vi "IMULoop.vi"   [LabVIEW 2015]
uses:
  Common Code/IMU Data.ctl
  Robot Global Data.vi
  navX-MXP Library/navX-MXP IMU.lvlib
  navX.Library.v2/navX Library v2/navX Library v2.lvlib
  navX.Library.v2/navX Library v2/TypeDefs/Flags/Z900_navX_Flags_OpStatusTypeDef.ctl
  navX.Library.v2/navX Library v2/TypeDefs/Flags/Z900_navX_Flags_CalibrationStatusTypeDef.ctl
types:
  T1 = typedef "IMU Data.ctl" = cluster{"Pitch":sgl, "Roll":sgl, "Yaw":sgl, "Data Valid?":bool, "Temp":sgl, "MOVING":bool, "YAW_STABLE":bool, "Accel X":sgl, "Accel Y":sgl, "Accel Z":sgl, "Accel Magnitude":sgl, "Pitch Rate":sgl, "Roll Rate":sgl, "Yaw Rate":sgl, "NavX Opened?":bool, "Calibration Status":T2, "OP Status":T3}
  T2 = typedef "navX Library v2.lvlib/Z900_navX_Flags_CalibrationStatusTypeDef.ctl" = u8
  T3 = typedef "navX Library v2.lvlib/Z900_navX_Flags_OpStatusTypeDef.ctl" = u8
  T4 = typedef "navX-MXP IMU.lvlib/navX Device TypeDef.ctl" = cluster{"navX Interface Protocol":T5, "navX Interface Protocol TypeDefs":cluster{"SPIDevRef":T6, "I2CDevRef":T8}, "navX System Information":cluster{"Board Information":T10, "Status":T11, "Offsets":T15}, "navX Common Information":cluster{"Update Rate (4Hz-60Hz)":T16, "refnum name":string, "error":errorcluster}}
  T5 = typedef "navX-MXP IMU.lvlib/navX Interface Protocol.ctl" = enum16{"SPI", "I2C"}
  T6 = typedef "WPI_SPIDevRef.ctl" = cluster{"DevStatus":errorcluster, "Handle":i32, "SPI Bus":T7}
  T7 = typedef "spi_bus.ctl" = enum16{"SPI On-Board, CS0", "SPI On-Board, CS1", "SPI On-Board, CS2", "SPI On-Board, CS3", "SPI MXP", "Invalid"}
  T8 = typedef "WPI_I2CDevRef.ctl" = cluster{"DevStatus":errorcluster, "Device Address":u8, "Handle":i32, "I2C Bus":T9}
  T9 = typedef "i2c_bus.ctl" = enum16{"I2C On-Board", "I2C MXP", "Invalid"}
  T10 = typedef "navX-MXP IMU.lvlib/navX Board Information.ctl" = cluster{"WhoAmI (50 | 0x32)":u8, "Board Revision":u8, "Firmware Major Version":u8, "Firmware Minor Version":u8}
  T11 = typedef "navX-MXP IMU.lvlib/navX Status Data.ctl" = cluster{"Update Rate Hz":u8, "Accelerometer Full-Scale Range":u8, "Gyro Full-Scale Range":u16, "NAVX_OP_STATUS":T12, "NAVX_CAL_STATUS":T13, "NAVX_SELFTEST_STATUS":u8, "NAVX_SENSOR_STATUS":T14}
  T12 = typedef "navX-MXP IMU.lvlib/navX NAVX_OP_STATUS.ctl" = u8
  T13 = typedef "navX-MXP IMU.lvlib/navX NAVX_CAL_STATUS.ctl" = u8
  T14 = typedef "navX-MXP IMU.lvlib/navX NAVX_SENSOR_STATUS.ctl" = cluster{"MOVING":bool, "YAW_STABLE":bool, "MAG_DISTURBANCE":bool, "ALTITUDE_VALID":bool, "SEALEVEL_PRESS_SET":bool, "FUSED_HEADING_VALID":bool}
  T15 = typedef "navX-MXP IMU.lvlib/navX Offsets Data.ctl" = cluster{"Yaw":dbl, "Quat W":dbl, "Quat X":dbl, "Quat Y":dbl, "Quat Z":dbl}
  T16 = typedef "navX-MXP IMU.lvlib/navX Update Rate.ctl" = u8
  T17 = typedef "navX-MXP IMU.lvlib/navX Vector Data.ctl" = cluster{"X":dbl, "Y":dbl, "Z":dbl}
  T18 = typedef "navX-MXP IMU.lvlib/navX YPRH Data.ctl" = cluster{"Yaw":dbl, "Pitch":dbl, "Roll":dbl, "Heading":dbl}
  T19 = typedef "navX Library v2.lvlib/Z900_navX_DeviceTypeDef.ctl" = cluster{"Interface":cluster{"Protocol":T20, "Update Rate (4Hz-60Hz)":u8, "navX Open TypeDef":variant}, "Notify Packet":refnum<notifier>, "Loop VI Refnum":refnum<vi>, "Ready to Close Occurrence Refnum":refnum<k4>}
  T20 = typedef "navX Library v2.lvlib/Z900_navX_ProtocolTypeDef.ctl" = enum16{"SERIAL", "I2C", "SPI"}
  T21 = cluster{"Accel X":dbl, "Accel Y":dbl, "Accel Z":dbl, "Gyro X":dbl, "Gyro Y":dbl, "Gyro Z":dbl, "Mag X":dbl, "Mag Y":dbl, "Mag Z":dbl}
  T22 = cluster{"Yaw":dbl, "Roll":dbl, "Pitch":dbl, "Heading":dbl, "Fused Heading":dbl}
  T23 = cluster{"Update Rate Hz":u8, "Accelerometer Full-Scale Range":u8, "Gyro Full-Scale Range":u16, "OP Status":T3, "Calibration Status":T2, "Sensor Status":cluster{"MOVING":bool, "YAW_STABLE":bool, "MAG_DISTURBANCE":bool, "ALTITUDE_VALID":bool, "SEALEVEL_PRESS_SET":bool, "FUSED_HEADING_VALID":bool}, "Self Test Status":cluster{"Gyro Passed":bool, "Accel Passed":bool, "Mag Passed":bool, "Baro Passed":bool, "Complete":bool}}
  T24 = cluster{"LinearAcceleration X":dbl, "LinearAcceleration Y":dbl, "LinearAcceleration Z":dbl}
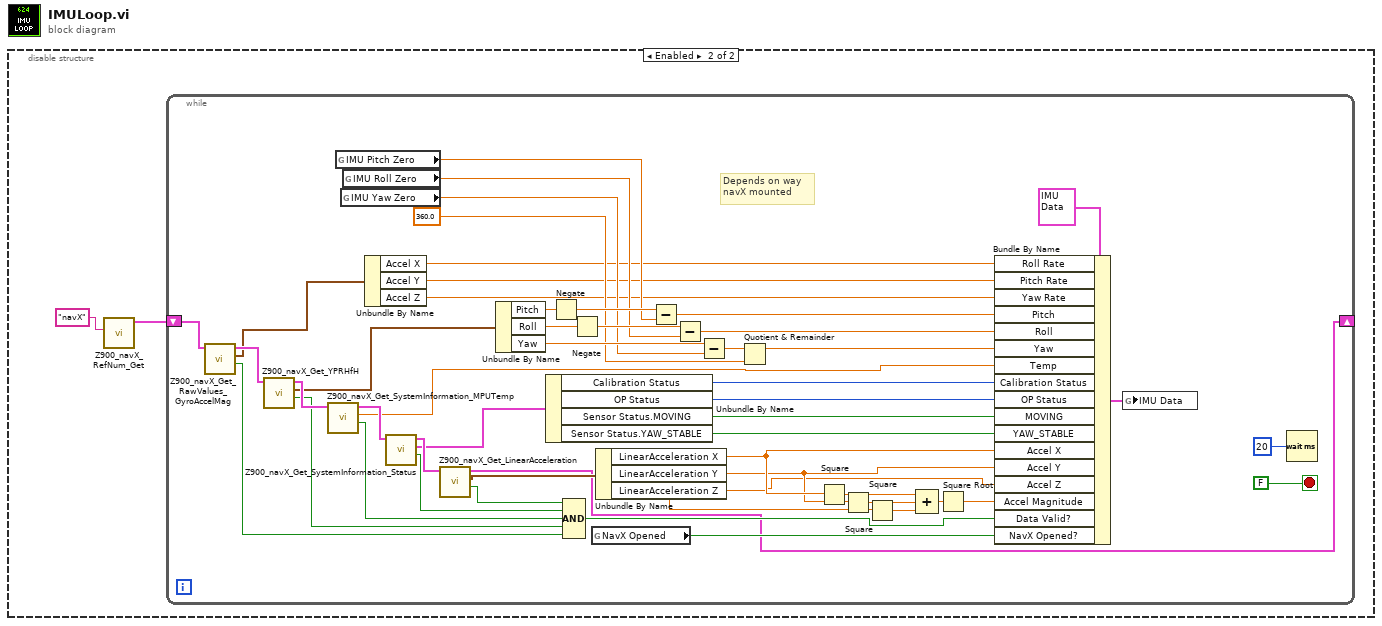
[diagram p0: block diagram]
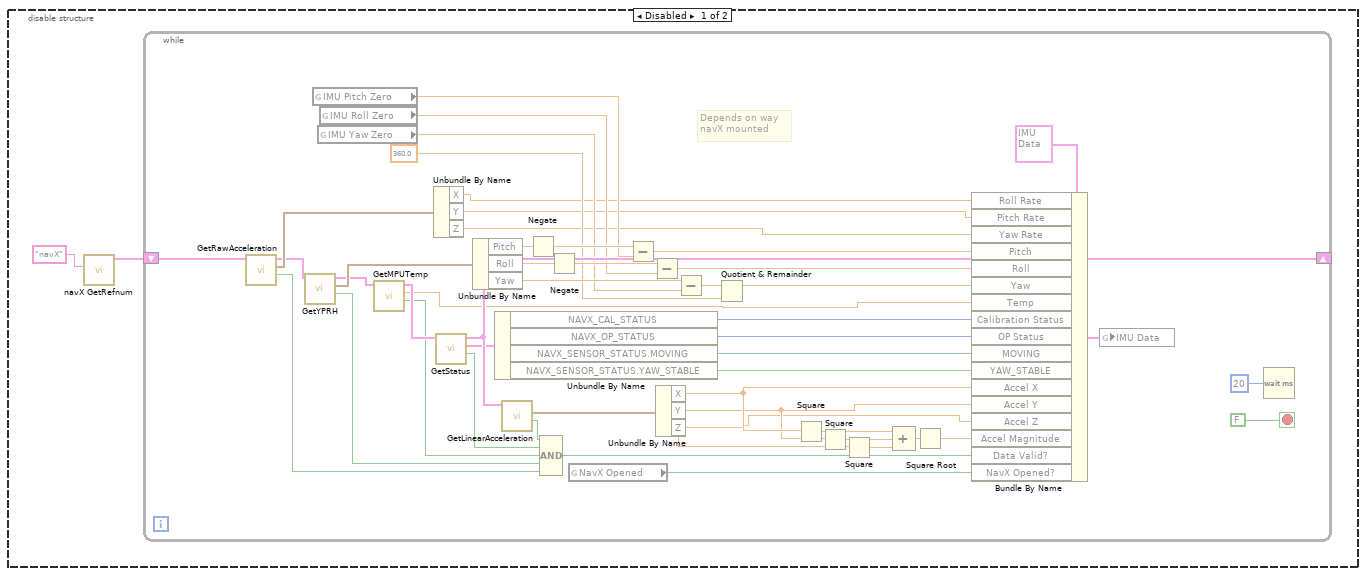
[diagram p2: hidden frame]
diagram:
  n1 = disable-structure shown="Enabled" {
    frame Disabled {
      n2 = call "navX GetRefnum.vi"("refnum name"="navX") -> ("navX Device TypeDef"=w1:T4)  [unwired: 9 in, 1 out]
      n3 = while {
        shift-right: [w48] -> _
        shift-left: w1 -> [w49]
        stop <- FALSE stop-if-true
        # "Depends on way \nnavX mounted"
        n4 = call "GetRawAcceleration.vi"("navX Device TypeDef"=w49) -> ("Valid?"=w17:bool, "Raw Acceleration"=w18:T17, "navX Device TypeDef"=w16:T4)  [unwired: 8 in]
        n5 = call "GetYPRH.vi"("navX Device TypeDef"=w16) -> ("Valid?"=w14:bool, "YPRH"=w15:T18, "navX Device TypeDef"=w13:T4)  [unwired: 8 in]
        n6 = global read "Robot Global Data.vi" "IMU Pitch Zero"() -> (w40:dbl)
        n7 = global read "Robot Global Data.vi" "IMU Yaw Zero"() -> (w38:dbl)
        n8 = global read "Robot Global Data.vi" "IMU Roll Zero"() -> (w39:dbl)
        n9 = call "GetMPUTemp.vi"("navX Device TypeDef"=w13) -> ("Valid?"=w6:bool, "MPU Temperature (Centigrade)"=w7:dbl, "navX Device TypeDef"=w12:T4)  [unwired: 8 in]
        n10 = Unbundle By Name(w18) -> ("X"=w5:dbl, "Y"=w4:dbl, "Z"=w3:dbl)
        n11 = call "GetStatus.vi"("navX Device TypeDef"=w12) -> ("Valid?"=w11:bool, "Status"=w8:T11, "navX Device TypeDef"=w48:T4)  [unwired: 8 in]
        n12 = Unbundle By Name(w15) -> ("Pitch"=w45:dbl, "Roll"=w44:dbl, "Yaw"=w41:dbl)
        n13 = Unbundle By Name(w8) -> ("NAVX_CAL_STATUS"=w22:T13, "NAVX_OP_STATUS"=w21:T12, "NAVX_SENSOR_STATUS.MOVING"=w20:bool, "NAVX_SENSOR_STATUS.YAW_STABLE"=w19:bool)
        n14 = call "GetLinearAcceleration.vi"("navX Device TypeDef"=w48) -> ("Valid?"=w10:bool, "Linear Acceleration"=w9:T17)  [unwired: 8 in, 1 out]
        n15 = Negate(x=w45) -> (-x=w43:dbl)
        n16 = Compound Arithmetic op=AND(w10, w11, w6, w14, w17) -> (w33:bool)
        n17 = Negate(x=w44) -> (-x=w42:dbl)
        n18 = global read "Robot Global Data.vi" "NavX Opened"() -> (w31:bool)
        n19 = Subtract(x=w43, y=w40) -> (x-y=w37:dbl)
        n20 = Subtract(x=w42, y=w39) -> (x-y=w36:dbl)
        n21 = Unbundle By Name(w9) -> ("X"=w25:dbl, "Y"=w24:dbl, "Z"=w23:dbl)
        n22 = Subtract(x=w41, y=w38) -> (x-y=w35:dbl)
        n23 = Quotient & Remainder(x=w35, y=360.0) -> (x-y*floor(x/y)=w34:dbl)  [unwired: 1 out]
        n24 = Square(x=w25) -> (x^2=w30:dbl)
        n25 = Square(x=w24) -> (x^2=w29:dbl)
        n26 = Square(x=w23) -> (x^2=w28:dbl)
        n27 = Compound Arithmetic op=ADD(w30, w29, w28) -> (w27:dbl)
        n28 = Square Root(x=w27) -> (sqrt(x)=w26:dbl)
        n29 = Bundle By Name(cluster=T1 {"Pitch"=0.0, "Roll"=0.0, "Yaw"=0.0, "Data Valid?"=FALSE, "Temp"=0.0, "MOVING"=FALSE, "YAW_STABLE"=FALSE, "Accel X"=0.0, "Accel Y"=0.0, "Accel Z"=0.0, "Accel Magnitude"=0.0, "Pitch Rate"=0.0, "Roll Rate"=0.0, "Yaw Rate"=0.0, "NavX Opened?"=FALSE, "Calibration Status"=0, "OP Status"=0} ("IMU Data"), "Roll Rate"=w5, "Pitch Rate"=w4, "Yaw Rate"=w3, "Pitch"=w37, "Roll"=w36, "Yaw"=w34, "Temp"=w7, "Calibration Status"=w22, "OP Status"=w21, "MOVING"=w20, "YAW_STABLE"=w19, "Accel X"=w25, "Accel Y"=w24, "Accel Z"=w23, "Accel Magnitude"=w26, "Data Valid?"=w33, "NavX Opened?"=w31) -> (w46:T1)
        n30 = global write "Robot Global Data.vi" "IMU Data"(w46) -> ()
        n31 = Wait (ms)(milliseconds to wait=u32 20) -> ()  [unwired: 1 out]
      }
    }
    frame Enabled {
      n32 = call "Z900_navX_RefNum_Get.vi"("refnum name"="navX") -> ("navX Device"=w52:T19)  [unwired: 9 in, 1 out]
      n33 = while {
        shift-right: [w54] -> _
        shift-left: w52 -> [w70]
        stop <- FALSE stop-if-true
        # "Depends on way \nnavX mounted"
        n34 = call "Z900_navX_Get_RawValues_GyroAccelMag.vi"("navX Device"=w70) -> ("Connected"=w65:bool, "Raw Values"=w55:T21, "navX Device"=w69:T19)  [unwired: 7 in, 1 out]
        n35 = call "Z900_navX_Get_YPRHfH.vi"("navX Device"=w69) -> ("Connected"=w64:bool, "YRPHfH"=w56:T22, "navX Device"=w68:T19)  [unwired: 7 in, 1 out]
        n36 = call "Z900_navX_Get_SystemInformation_MPUTemp.vi"("navX Device"=w68) -> ("Connected"=w63:bool, "MPUTemp"=w57:dbl, "navX Device"=w67:T19)  [unwired: 7 in, 1 out]
        n37 = global read "Robot Global Data.vi" "IMU Pitch Zero"() -> (w94:dbl)
        n38 = global read "Robot Global Data.vi" "IMU Yaw Zero"() -> (w92:dbl)
        n39 = global read "Robot Global Data.vi" "IMU Roll Zero"() -> (w93:dbl)
        n40 = Unbundle By Name(w55) -> ("Accel X"=w73:dbl, "Accel Y"=w72:dbl, "Accel Z"=w71:dbl)
        n41 = call "Z900_navX_Get_SystemInformation_Status.vi"("navX Device"=w67) -> ("Connected"=w62:bool, "Status"=w58:T23, "navX Device"=w66:T19)  [unwired: 7 in, 1 out]
        n42 = call "Z900_navX_Get_LinearAcceleration.vi"("navX Device"=w66) -> ("Connected"=w61:bool, "Linear Acceleration"=w60:T24, "navX Device"=w54:T19)  [unwired: 7 in, 1 out]
        n43 = Unbundle By Name(w56) -> ("Pitch"=w99:dbl, "Roll"=w98:dbl, "Yaw"=w95:dbl)
        n44 = Unbundle By Name(w58) -> ("Calibration Status"=w77:T2, "OP Status"=w76:T3, "Sensor Status.MOVING"=w75:bool, "Sensor Status.YAW_STABLE"=w74:bool)
        n45 = Negate(x=w99) -> (-x=w97:dbl)
        n46 = Compound Arithmetic op=AND(w61, w62, w63, w64, w65) -> (w59:bool)
        n47 = Negate(x=w98) -> (-x=w96:dbl)
        n48 = global read "Robot Global Data.vi" "NavX Opened"() -> (w86:bool)
        n49 = Unbundle By Name(w60) -> ("LinearAcceleration X"=w80:dbl, "LinearAcceleration Y"=w79:dbl, "LinearAcceleration Z"=w78:dbl)
        n50 = Subtract(x=w97, y=w94) -> (x-y=w91:dbl)
        n51 = Subtract(x=w96, y=w93) -> (x-y=w90:dbl)
        n52 = Subtract(x=w95, y=w92) -> (x-y=w89:dbl)
        n53 = Quotient & Remainder(x=w89, y=360.0) -> (x-y*floor(x/y)=w88:dbl)  [unwired: 1 out]
        n54 = Square(x=w80) -> (x^2=w85:dbl)
        n55 = Square(x=w79) -> (x^2=w84:dbl)
        n56 = Square(x=w78) -> (x^2=w83:dbl)
        n57 = Compound Arithmetic op=ADD(w85, w84, w83) -> (w82:dbl)
        n58 = Square Root(x=w82) -> (sqrt(x)=w81:dbl)
        n59 = Bundle By Name(cluster=T1 {"Pitch"=0.0, "Roll"=0.0, "Yaw"=0.0, "Data Valid?"=FALSE, "Temp"=0.0, "MOVING"=FALSE, "YAW_STABLE"=FALSE, "Accel X"=0.0, "Accel Y"=0.0, "Accel Z"=0.0, "Accel Magnitude"=0.0, "Pitch Rate"=0.0, "Roll Rate"=0.0, "Yaw Rate"=0.0, "NavX Opened?"=FALSE, "Calibration Status"=0, "OP Status"=0} ("IMU Data"), "Roll Rate"=w73, "Pitch Rate"=w72, "Yaw Rate"=w71, "Pitch"=w91, "Roll"=w90, "Yaw"=w88, "Temp"=w57, "Calibration Status"=w77, "OP Status"=w76, "MOVING"=w75, "YAW_STABLE"=w74, "Accel X"=w80, "Accel Y"=w79, "Accel Z"=w78, "Accel Magnitude"=w81, "Data Valid?"=w59, "NavX Opened?"=w86) -> (w100:T1)
        n60 = global write "Robot Global Data.vi" "IMU Data"(w100) -> ()
        n61 = Wait (ms)(milliseconds to wait=u32 20) -> ()  [unwired: 1 out]
      }
    }
  }
